vi "Move Menu Down.vi"(8 "error in (no error)":errorcluster, 11 "Display State In":T1={"Numeric"=0.0, "Array of Button References"=[], "Space Between Menu Buttons"=0, "Number of Menu Buttons"=0, "Array of Button Names"=[], "Most Recent Vertical Position"=0, "This VI"=refnum, "Current Action"=enum."Not Moving", "Most Recent Distance Traveled"=0, "Method"=enum."Move Up", "Data In"=0} caption="State") -> (0 "error out":errorcluster, 3 "Display State Out":T1={"Numeric"=0.0, "Array of Button References"=[], "Space Between Menu Buttons"=0, "Number of Menu Buttons"=0, "Array of Button Names"=[], "Most Recent Vertical Position"=0, "This VI"=refnum, "Current Action"=enum."Not Moving", "Most Recent Distance Traveled"=0, "Method"=enum."Move Up", "Data In"=0} caption="State")   [LabVIEW 2011, in "Sliding Menu Library.lvlib" / "Sliding Menu XControl.xctl"]
uses:
  Sliding Menu XControl.xctl
  Sliding Menu State.ctl
  Menu Button Library/Menu Button xControl/Menu Button xControl.xctl
  Sliding Menu SubVIs/Sliding Menu Type Definitions/Current User Action.ctl
  Sliding Menu Methods.ctl
  Sliding Menu Data.ctl
  Sliding Menu Library.lvlib
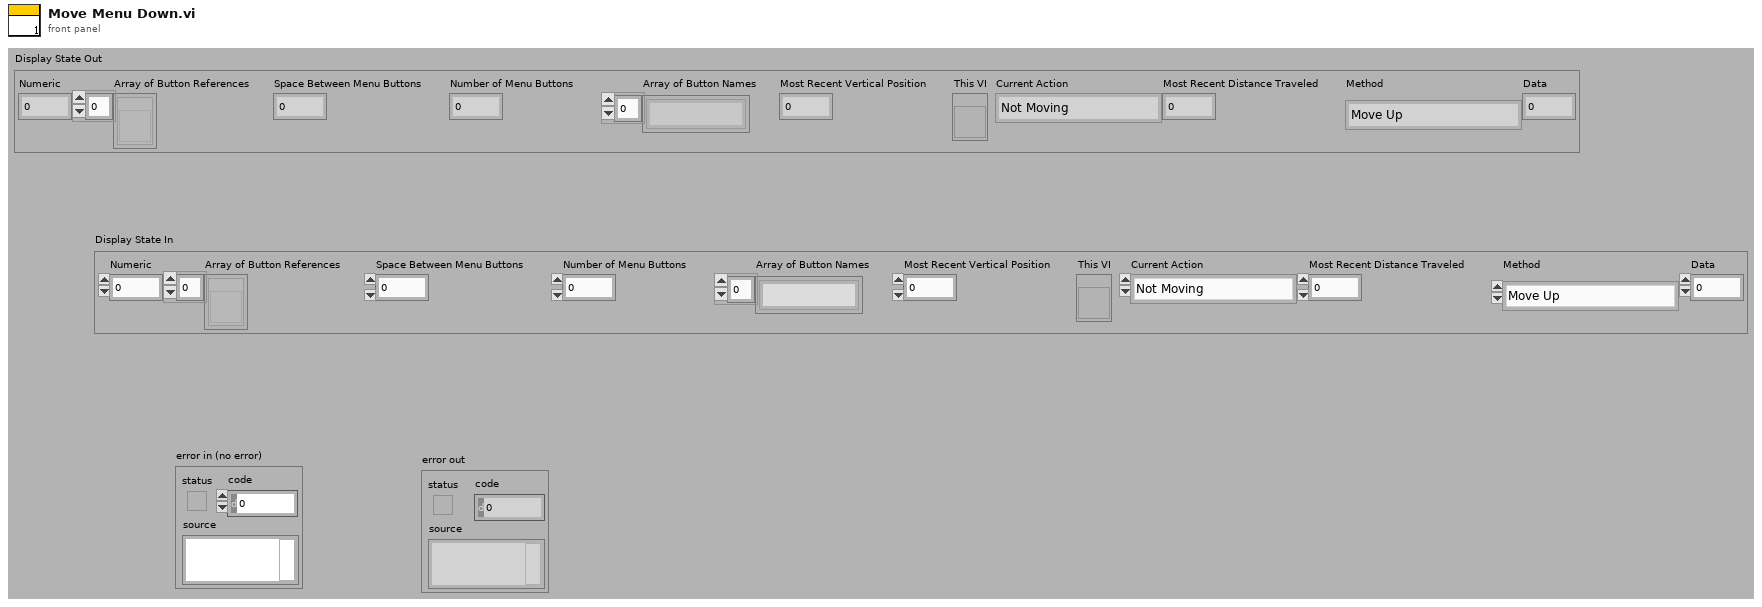
[diagram p1: front panel]
types:
  T1 = typedef "Sliding Menu Library.lvlib/Sliding Menu XControl.xctl/Sliding Menu State.ctl" = cluster{"Numeric":dbl, "Array of Button References":refnum<vi>[], "Space Between Menu Buttons":i32, "Number of Menu Buttons":i32, "Array of Button Names":string[], "Most Recent Vertical Position":i32, "This VI":refnum<vi>, "Current Action":T2, "Most Recent Distance Traveled":i32, "Method":T3, "Data In":T4}
  T2 = typedef "Sliding Menu Library.lvlib/Current User Action.ctl" = enum16{"Not Moving", "Mouse Down", "Mouse Up No Dragging", "Bounce Up Needed", "Bounce Down Needed", "Dragging", "Easing"}
  T3 = typedef "Sliding Menu Methods.ctl" = enum16{"Resize", "Move Up", "Move Down", "Move to 0"}
  T4 = typedef "Sliding Menu Library.lvlib/Sliding Menu XControl.xctl/Sliding Menu Data.ctl" = i32
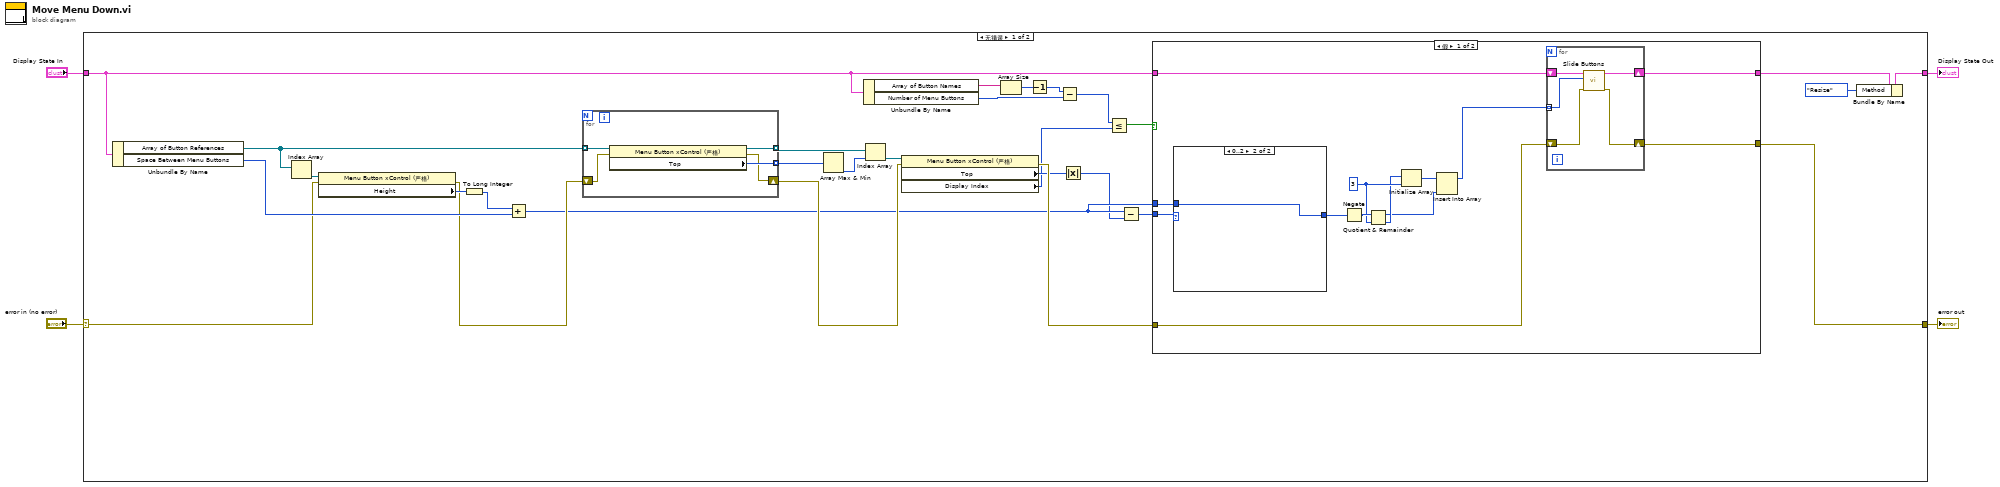
[diagram p0: block diagram]
diagram:
  n1 = case shown="无错误" "error in (no error)" {
    selector: "error in (no error)" -> [w20 w62]
    tunnel: [w33 w62] -> w4
    tunnel: "Display State In" -> [w12 w61]
    tunnel: [w31 w61] -> w1
    frame No Error {
      n2 = Unbundle By Name(w12) -> ("Array of Button References"=w26:refnum<vi>[], "Space Between Menu Buttons"=w23:i32)
      n3 = Index Array(array=w26) -> (element=w25:refnum<vi>)  [unwired: 1 in]
      n4 = property class="Menu Button xControl (严格)"(reference=w25, error in=w20) -> (error out=w19:errorcluster, "Height"=w22:u32)  [unwired: 1 out]
      n5 = To Long Integer(number=w22) -> (32bit integer=w21:i32)
      n6 = Add(x=w21, y=w23) -> (x+y=w14:i32)
      n7 = for {
        tunnel: w26 -> [w60] mode=indexing
        tunnel: [w59] -> w29 mode=indexing
        tunnel: [w58] -> w28 mode=indexing
        shift-right: [w57] -> w18
        shift-left: w19 -> [w56]
        n8 = property class="Menu Button xControl (严格)"(reference=w60, error in=w56) -> (reference out=w58:refnum<vi>, error out=w57:errorcluster, "Top"=w59:i32)
      }
      n9 = Array Max & Min(array=w29) -> (min index (indices)=w27:i32)  [unwired: 3 out]
      n10 = Unbundle By Name(w12) -> ("Array of Button Names"=w11:string[], "Number of Menu Buttons"=w8:i32)
      n11 = Index Array(array=w28, index=w27) -> (element=w24:refnum<vi>)
      n12 = property class="Menu Button xControl (严格)"(reference=w24, error in=w18) -> (error out=w17:errorcluster, "Top"=w16:i32, "Display Index"=w6:i32)  [unwired: 1 out]
      n13 = Array Size(array=w11) -> (size(s)=w10:i32)
      n14 = Decrement(x=w10) -> (x-1=w9:i32)
      n15 = Subtract(x=w9, y=w8) -> (x-y=w7:i32)
      n16 = Absolute Value(x=w16) -> (abs(x)=w13:i32)
      n17 = Less Or Equal?(x=w7, y=w6) -> (x <= y?=w5:bool)
      n18 = Subtract(x=w14, y=w13) -> (x-y=w15:i32)
      n19 = case shown="假" w5 {
        tunnel: [w46 w54] -> w33
        tunnel: [w45 w55] -> w32
        tunnel: w12 -> [w44 w55]
        tunnel: w17 -> [w43 w54]
        tunnel: w15 -> [w36 _]
        tunnel: w14 -> [w34 _]
        frame False {
          w41 = 3 ("y")
          n20 = case shown="0..2" w36 {
            selector: w36 -> [w47 _]
            tunnel: [w47 w48] -> w35
            tunnel: w34 -> [_ w48]
            frame Default {
            }
            frame 0..2 {
            }
          }
          n21 = Negate(x=w35) -> (-x=w42:i32)
          n22 = Quotient & Remainder(x=w42, y=w41) -> (x-y*floor(x/y)=w37:i32, floor(x/y)=w38:i32)
          n23 = Initialize Array(w38, w41) -> (w40:i32[])
          n24 = Insert Into Array(array=w40, new element=w37) -> (w39:i32[])  [unwired: 1 in]
          n25 = for {
            shift-right: [w52] -> w45
            shift-left: w44 -> [w51]
            shift-right: [w53] -> w46
            shift-left: w43 -> [w50]
            tunnel: w39 -> [w49] mode=indexing
            n26 = call "Slide Buttons.vi"("error in (no error)"=w50, "Distance"=w49, "Display State In"=w51) -> ("error out"=w53:errorcluster, "Display State Out"=w52:T1)  [unwired: 7 in]
          }
        }
        frame True {
        }
      }
      n27 = Bundle By Name(cluster=w32, "Method"=Sliding_Menu_Methods."Resize") -> (w31:T1)
    }
    frame Error {
    }
  }
  "error out" <- w4
  "Display State Out" <- w1
